vi "_API_BINANCE_GET_Ping.vi"(0 "BinanceAPI in":refnum<class "BinanceAPI_.lvclass">, 11 "error in (no error)":errorcluster) -> (4 "BinanceAPI out":refnum<class "BinanceAPI_.lvclass">, 6 "Is Binance Work?":bool, 14 "Data":string, 15 "error out":errorcluster)   [LabVIEW 2022 SP3, in "BinanceAPI_.lvclass"]
doc: "Ping Binance API and if response is: \"{}\" the \"Is Binance Work?\" indicator show \"True\"\n\nhttps://binance-docs.github.io/apidocs/spot/en/#test-connectivity"
uses:
  BinanceAPI_.lvclass
  BinanceAPI_.lvclass/BinanceAPI_.ctl
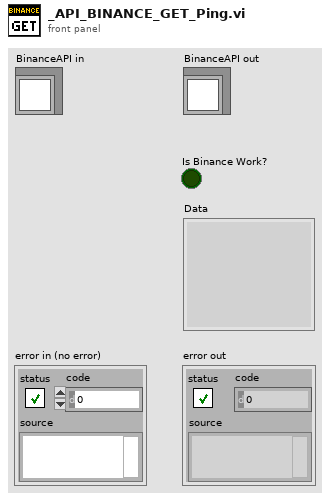
[diagram p1: front panel]
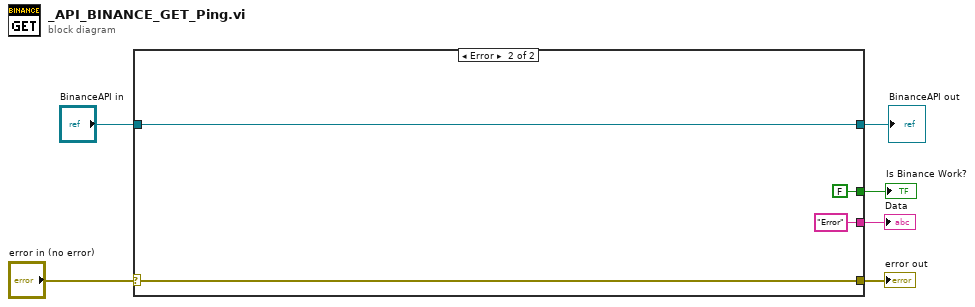
[diagram p0: block diagram]
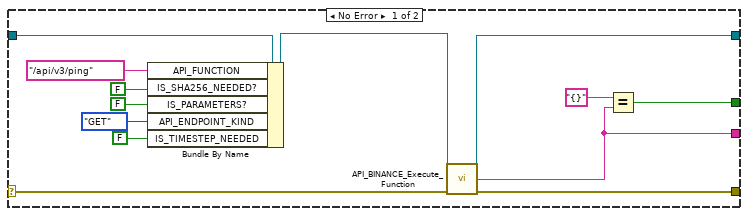
[diagram p2: hidden frame]
diagram:
  n1 = case shown="Error" "error in (no error)" {
    selector: "error in (no error)" -> [w12 w23]
    tunnel: [w11 w23] -> w5
    tunnel: [w13 w22] -> w1
    tunnel: "BinanceAPI in" -> [w15 w22]
    tunnel: [w8 "Error" ("Dane")] -> w4
    tunnel: [w7 FALSE] -> w3
    frame No Error {
      n2 = Bundle By Name(cluster=w15, "API_FUNCTION"="/api/v3/ping", "IS_SHA256_NEEDED?"=FALSE, "IS_PARAMETERS?"=FALSE, "API_ENDPOINT_KIND"=enum16{"POST", "DELETE", "GET", "PUT"}."GET", "IS_TIMESTEP_NEEDED"=FALSE) -> (w14:refnum<class "BinanceAPI_.lvclass">)
      n3 = call "API_BINANCE_Execute_Function.vi"("BinanceAPI in"=w14, "error in (no error)"=w12) -> ("BinanceAPI out"=w13:refnum<class "BinanceAPI_.lvclass">, "Body"=w8:string, "error out"=w11:errorcluster)  [unwired: 9 in, 2 out]
      n4 = Equal?(x="{}" ("Body"), y=w8) -> (x = y?=w7:bool)
    }
    frame Error {
    }
  }
  "error out" <- w5
  "Data" <- w4
  "Is Binance Work?" <- w3
  "BinanceAPI out" <- w1
